vi "Generic command handler.vi"(8 "error in (no error)":errorcluster, 10 "Message in":refnum<class "GenericMessage.lvclass">, 11 "RSA in":refnum<class "RSA.lvclass">) -> (0 "error out":errorcluster, 2 "command":string, 3 "RSA out":refnum<class "RSA.lvclass">)   [LabVIEW 2012, in "RSA.lvclass"]
doc: "The generic_command_handler processes the command 'generic'. Commands which are not part of the predefined list of commands fall under the 'generic' command for special activity."
uses:
  RSA.lvclass
  <vilib>/Distrio/Murmex/GenericMessage/GenericMessage.lvclass
  <vilib>/Distrio/Murmex/Murmex/Murmex.lvclass
  RSA.lvclass/RSA.ctl
  <vilib>/Distrio/Murmex/ProceedMessage/ProceedMessage.lvclass
  <vilib>/Analysis/NI_AALBase.lvlib
  <vilib>/Distrio/Murmex/Message/Message.lvclass
panel:
  # "This method is called when the GENERIC\ntrigger is sent. \n\nOverride this method when your component needs to\nrespond to this trigger. \n\nCall parent for proper implementation"
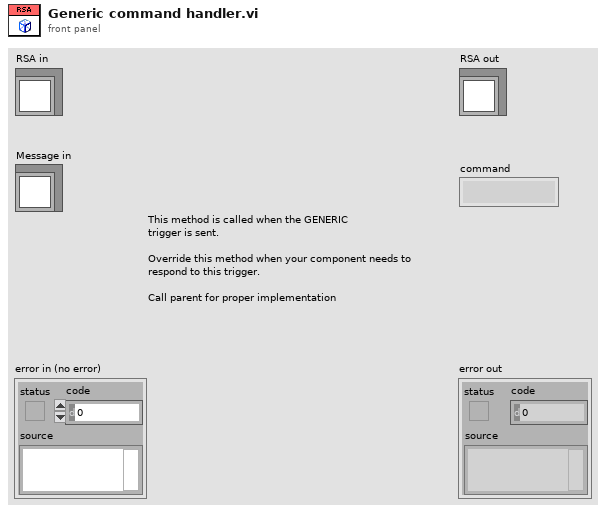
[diagram p1: front panel]
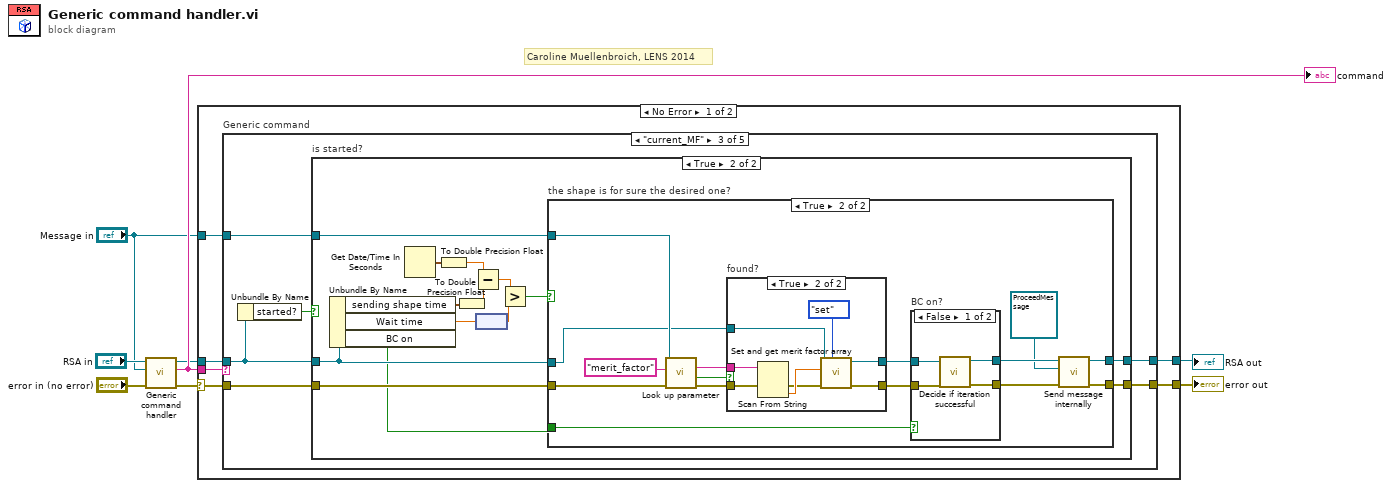
[diagram p0: block diagram]
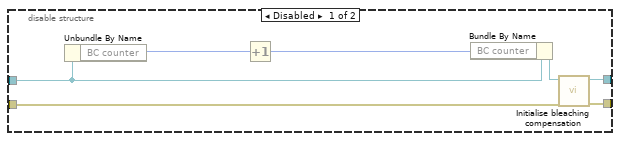
[diagram p4: hidden frame]
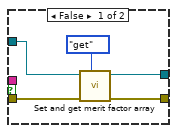
[diagram p8: hidden frame]
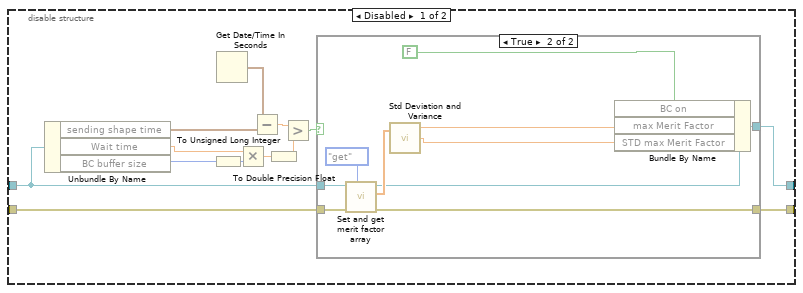
[diagram p10: hidden frame]
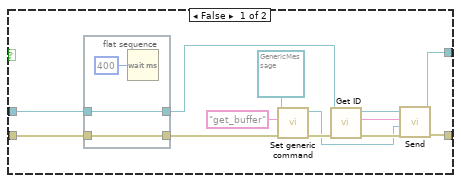
[diagram p11: hidden frame]
diagram:
  # "Caroline Muellenbroich, LENS 2014"
  n1 = call-parent "Generic command handler.vi"("error in (no error)"="error in (no error)", "Message in"="Message in", "Murmex in"="RSA in") -> ("error out"=w6:errorcluster, "value"=w5:string, "Murmex out"=w3:refnum<class "RSA.lvclass">)  [unwired: 6 in]
  "command" <- w5
  n2 = case shown="No Error" w6 {
    selector: w6 -> [w14 w136]
    tunnel: w5 -> [w13 _]
    tunnel: [w12 w136] -> w4
    tunnel: w3 -> [w11 w135]
    tunnel: [w10 w135] -> w2
    tunnel: "Message in" -> [w9 _]
    frame No Error {
      n3 = case "Generic command" shown="\"current_MF\"" w13 {
        tunnel: w14 -> [w16 w20 w35 w91 w133]
        tunnel: [w16 w19 w34 w90 w133] -> w12
        tunnel: w11 -> [w15 w18 w31 w88 w134]
        tunnel: [w15 w17 w33 w89 w134] -> w10
        tunnel: w9 -> [_ _ w32 _ _]
        frame "False", Default {
        }
        frame "bleaching_on" {
          n4 = disable-structure shown="Enabled" {
            disable-tunnel: w20 -> [w27 w28]
            disable-tunnel: [w26 w28] -> w19
            disable-tunnel: w18 -> [w25 w29]
            disable-tunnel: [w23 w29] -> w17
            frame Disabled {
              n5 = Unbundle By Name(w25) -> ("BC counter"=w22:i32)
              n6 = Increment(x=w22) -> (x+1=w21:i32)
              n7 = Bundle By Name(cluster=w25, "BC counter"=w21) -> (w24:refnum<class "RSA.lvclass">)
              n8 = call-dynamic "Initialise bleaching compensation.vi"("error in (no error)"=w27, "RSA in"=w24) -> ("error out"=w26:errorcluster, "RSA out"=w23:refnum<class "RSA.lvclass">)  [unwired: 8 in]
            }
            frame Enabled {
            }
          }
        }
        frame "current_MF" {
          n9 = Unbundle By Name(w31) -> ("started?"=w30:bool)
          n10 = case "is started?" shown="True" w30 {
            tunnel: w35 -> [w36 w51]
            tunnel: [w36 w50] -> w34
            tunnel: [w37 w49] -> w33
            tunnel: w31 -> [w37 w48]
            tunnel: w32 -> [_ w45]
            frame False {
            }
            frame True {
              n11 = Unbundle By Name(w48) -> ("sending shape time"=w39:timestamp, "Wait time"=w43:dbl[unit], "BC on"=w44:bool)
              n12 = Get Date/Time In Seconds() -> (seconds since 1Jan1904=w41:timestamp)
              n13 = To Double Precision Float(number=w41) -> (double precision float=w40:dbl)
              n14 = To Double Precision Float(number=w39) -> (double precision float=w38:dbl)
              n15 = Subtract(x=w40, y=w38) -> (x-y=w47:dbl)
              n16 = node(w43) -> (w42:dbl)
              n17 = Greater?(x=w47, y=w42) -> (0:w46:bool)
              n18 = case "the shape is for sure the desired one?" shown="True" w46 {
                tunnel: w51 -> [w52 w62]
                tunnel: [w52 w68] -> w50
                tunnel: [w53 w67] -> w49
                tunnel: w48 -> [w53 w56]
                tunnel: w45 -> [_ w63]
                tunnel: w44 -> [_ w54]
                frame False {
                }
                frame True {
                  n19 = call <vilib>:"Look up parameter.vi"("error in (no error)"=w62, "name"="merit_factor", "Message in"=w63) -> ("error out"=w60:errorcluster, "found?"=w58:bool, "key"=w59:string)  [unwired: 5 in, 1 out]
                  n20 = case "found?" shown="True" w58 {
                    tunnel: w60 -> [w79 w87]
                    tunnel: [w78 w83] -> w57
                    tunnel: w59 -> [_ w86]
                    tunnel: w56 -> [w77 w82]
                    tunnel: [w76 w81] -> w55
                    frame False {
                      n21 = call "Set and get merit factor array.vi"("action"=enum16{"set", "get", "initialise"}."get", "error in (no error)"=w79, "RSA in"=w77) -> ("error out"=w78:errorcluster, "RSA out"=w76:refnum<class "RSA.lvclass">)  [unwired: 5 in, 2 out]
                    }
                    frame True {
                      n22 = Scan From String(input string=w86, error in=w87) -> (error out=w84:errorcluster, output 1=w85:dbl)  [unwired: 3 in, 2 out]
                      n23 = call "Set and get merit factor array.vi"("action"=enum16{"set", "get", "initialise"}."set", "error in (no error)"=w84, "merit factor"=w85, "RSA in"=w82) -> ("error out"=w83:errorcluster, "RSA out"=w81:refnum<class "RSA.lvclass">)  [unwired: 4 in, 2 out]
                    }
                  }
                  n24 = case "BC on?" shown="False" w54 {
                    tunnel: [w72 w73] -> w66
                    tunnel: [w71 w74] -> w65
                    tunnel: w57 -> [w70 w73]
                    tunnel: w55 -> [w69 w74]
                    frame False {
                      n25 = call-dynamic "Decide if iteration successful.vi"("error in (no error)"=w70, "RSA in"=w69) -> ("error out"=w72:errorcluster, "RSA out"=w71:refnum<class "RSA.lvclass">)  [unwired: 8 in]
                    }
                    frame True {
                    }
                  }
                  n26 = call <vilib>:"Send message internally.vi"("error in (no error)"=w66, "Message"=refnum<class "ProceedMessage.lvclass"> refnum ("ProceedMessage"), "Murmex in"=w65) -> ("error out"=w68:errorcluster, "Murmex out"=w67:refnum<class "RSA.lvclass">)  [unwired: 7 in]
                }
              }
            }
          }
        }
        frame "get_buffer" {
          n27 = disable-structure shown="Enabled" {
            disable-tunnel: w91 -> [w104 w131]
            disable-tunnel: [w103 w131] -> w90
            disable-tunnel: [w102 w132] -> w89
            disable-tunnel: w88 -> [w97 w132]
            frame Disabled {
              n28 = Unbundle By Name(w97) -> ("sending shape time"=w101:timestamp, "Wait time"=w95:dbl[unit], "BC buffer size"=w94:i32)
              n29 = To Unsigned Long Integer(number=w94) -> (unsigned 32bit integer=w93:u32)
              n30 = Get Date/Time In Seconds() -> (seconds since 1Jan1904=w100:timestamp)
              n31 = Multiply(x=w95, y=w93) -> (x*y=w96:dbl[unit])
              n32 = Subtract(x=w100, y=w101) -> (x-y=w99:dbl)
              n33 = To Double Precision Float(number=w96) -> (double precision float=w98:dbl[unit])
              n34 = Greater?(x=w99, y=w98) -> (0:w92:bool)
              n35 = case shown="True" w92 {
                tunnel: w104 -> [w107 w125]
                tunnel: [w106 w124] -> w103
                tunnel: [w105 w122] -> w102
                tunnel: w97 -> [w108 w121]
                frame False {
                  n36 = flat-sequence {
                    tunnel: [w119] -> w110
                    tunnel: w108 -> [w119]
                    tunnel: [w118] -> w109
                    tunnel: w107 -> [w118]
                    frame #0 {
                      n37 = Wait (ms)(milliseconds to wait=u32 400) -> ()  [unwired: 1 out]
                    }
                  }
                  n38 = call <vilib>:"Set generic command.vi"("error in (no error)"=w109, "generic command"="get_buffer", "GenericMessage in"=refnum<class "GenericMessage.lvclass"> refnum ("Distrio Murmex 1.5:GenericMessage")) -> ("error out"=w114:errorcluster, "GenericMessage out"=w111:refnum<class "GenericMessage.lvclass">)  [unwired: 7 in]
                  n39 = call <vilib>:"Get ID.vi"("error in (no error)"=w114, "Murmex in"=w110) -> ("error out"=w116:errorcluster, "component id"=w117:string, "Murmex out"=w115:refnum<class "RSA.lvclass">)  [unwired: 7 in]
                  n40 = call <vilib>:"Send.vi"("error in (no error)"=w116, "Message"=w111, "recipient"=w117, "Murmex in"=w115) -> ("error out"=w106:errorcluster, "Murmex out"=w105:refnum<class "RSA.lvclass">)  [unwired: 6 in]
                }
                frame True {
                  n41 = call "Set and get merit factor array.vi"("action"=enum16{"set", "get", "initialise"}."get", "error in (no error)"=w125, "RSA in"=w121) -> ("error out"=w124:errorcluster, "merit factor array"=w129:dbl[], "RSA out"=w123:refnum<class "RSA.lvclass">)  [unwired: 5 in, 1 out]
                  n42 = call <vilib>:"Std Deviation and Variance.vi"("X"=w129) -> ("mean"=w126:dbl, "standard deviation"=w127:dbl)  [unwired: 1 in, 1 out]
                  n43 = Bundle By Name(cluster=w123, "BC on"=FALSE ("Run time cluster.BC on"), "max Merit Factor"=w126, "STD max Merit Factor"=w127) -> (w122:refnum<class "RSA.lvclass">)
                }
              }
            }
            frame Enabled {
            }
          }
        }
        frame "dummy" {
        }
      }
    }
    frame Error {
    }
  }
  "error out" <- w4
  "RSA out" <- w2
